vi "ReadWrite Label.vi"(5 "Mode":T10, 6 "ScheduledSDI":bool, 7 "Iteration":i32, 8 "error in (no error)":errorcluster, 10 "FIFOs In":T1, 11 "Label In":T2 {"Driver Data"."Num Bits" min=1 max=32; "Driver Data"."Start Bit" min=8 max=31; "Block Data Refs"."Data Reference" format="%.0x"; "Label" format="%.0o"}) -> (0 "error out":errorcluster, 2 "FIFOs Out":T1, 3 "Label Out":T2 {"Driver Data"."Num Bits" min=1 max=32; "Driver Data"."Start Bit" min=8 max=31; "Block Data Refs"."Data Reference" format="%.0x"; "Label" format="%.0o"})   [LabVIEW 2011, in "AIT 1553 Custom Device.lvlib"]
uses:
  AIT 1553 Custom Device.lvlib
  RT Controls/ReadWrite Selector.ctl
  RT Controls/RT Label Settings.ctl
  Controls and Global/Label.ctl
  Controls and Global/transferPeriod.ctl
  <vilib>/NI Veristand/Custom Device API/Block Data Reference.ctl
  <vilib>/NI Veristand/Custom Device API/Data Reference.ctl
  RT Controls/Driver Data.ctl
  Controls and Global/Start Bit.ctl
  Controls and Global/Number of Bits.ctl
  RT Controls/FIFO.ctl
  Double to selected bits.vi
  SubVIs/Word to double.vi
  <vilib>/NI Veristand/Custom Device API/Global Data Refs.vi
  <instrlib>/AIT 429/Public/Tx/Data/AIT 429 Set Scheduled Label Datum.vi
  <instrlib>/AIT 429/Public/Tx/Data/AIT 429 Get Scheduled Label Datum.vi
  <vilib>/NI Veristand/Custom Device API/Custom Device API.lvlib
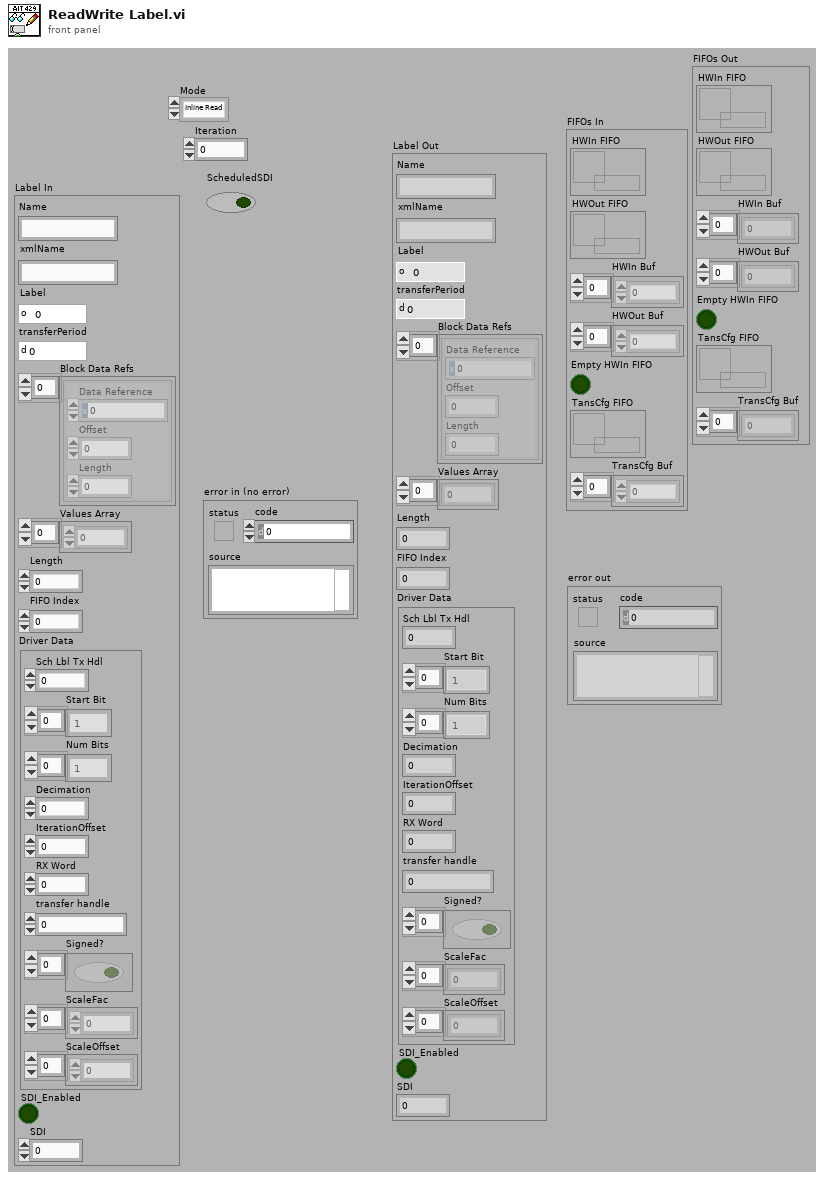
[diagram p1: front panel]
types:
  T1 = typedef "AIT 1553 Custom Device.lvlib/FIFO.ctl" = cluster{"HWIn FIFO":refnum<k33>, "HWOut FIFO":refnum<k33>, "HWIn Buf":dbl[], "HWOut Buf":dbl[], "Empty HWIn FIFO":bool, "TansCfg FIFO":refnum<k33>, "TransCfg Buf":dbl[]}
  T2 = typedef "AIT 1553 Custom Device.lvlib/RT Label Settings.ctl" = cluster{"Name":string, "xmlName":string, "Label":T3, "transferPeriod":T4, "Block Data Refs":T5[], "Values Array":dbl[], "Length":i32, "FIFO Index":i32, "Driver Data":T7, "SDI_Enabled":bool, "SDI":u8}
  T3 = typedef "AIT 1553 Custom Device.lvlib/Label.ctl" = u8
  T4 = typedef "AIT 1553 Custom Device.lvlib/transferPeriod.ctl" = u32
  T5 = typedef "Custom Device API.lvlib/Block Data Reference.ctl" = cluster{"Data Reference":T6, "Offset":i32, "Length":i32}
  T6 = typedef "Custom Device API.lvlib/Data Reference.ctl" = i32
  T7 = typedef "AIT 1553 Custom Device.lvlib/Driver Data.ctl" = cluster{"Sch Lbl Tx Hdl":u32, "Start Bit":T8[], "Num Bits":T9[], "Decimation":i32, "IterationOffset":i32, "RX Word":u32, "transfer handle":u32, "Signed?":bool[], "ScaleFac":dbl[], "ScaleOffset":dbl[]}
  T8 = typedef "AIT 1553 Custom Device.lvlib/Start Bit.ctl" = i32
  T9 = typedef "AIT 1553 Custom Device.lvlib/Number of Bits.ctl" = i32
  T10 = typedef "AIT 1553 Custom Device.lvlib/ReadWrite Selector.ctl" = enum16{"Inline Read", "Inline Write", "Async HWIn", "Async HWOut"}
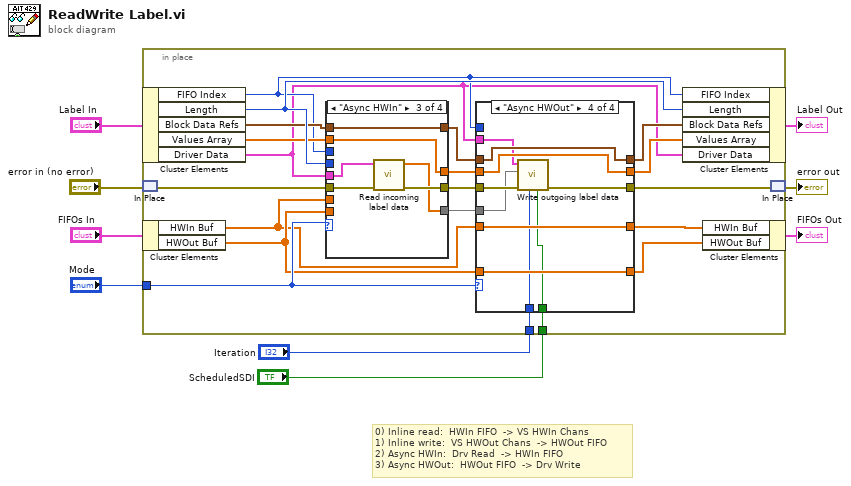
[diagram p0: block diagram]
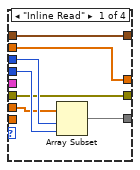
[diagram p2: hidden frame]
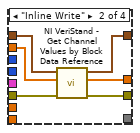
[diagram p3: hidden frame]
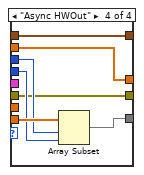
[diagram p4: hidden frame]
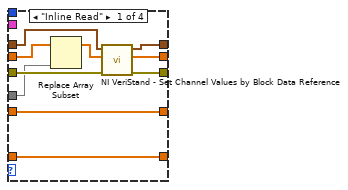
[diagram p5: hidden frame]
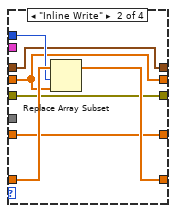
[diagram p6: hidden frame]
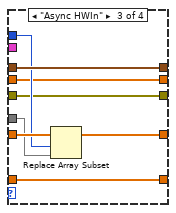
[diagram p7: hidden frame]
diagram:
  # "0) Inline read:\t\tHWIn FIFO \t-> VS HWIn Chans\n1) Inline write: \tVS HWOut Chans \t-> HWOut FIFO\n2) Async HWIn:\t\tDrv Read \t-> HWIn FIFO\n3) Async HWOut: \tHWOut FIFO \t-> Drv Write"
  n1 = in-place {
    in-place-border: "Mode" -> [w29]
    in-place-border: "Iteration" -> [w11]
    in-place-border: "ScheduledSDI" -> [w10]
    n2 = in-place-cluster #1("Label In") -> ("FIFO Index"=w16:i32, "Length"=w24:i32, "Block Data Refs"=w21:T5[], "Values Array"=w20:dbl[], "Driver Data"=w12:T7)
    n3 = in-place-match #2("error in (no error)") -> (w23:errorcluster)
    n4 = in-place-cluster #3("FIFOs In") -> ("HWIn Buf"=w13:dbl[], "HWOut Buf"=w14:dbl[])
    n5 = case shown="\"Async HWIn\"" w29 {
      tunnel: w13 -> [w33 _ _ _]
      tunnel: w16 -> [w36 _ _ w54]
      tunnel: w24 -> [w35 _ _ w53]
      tunnel: [w34 _ w43 w49] -> w28
      tunnel: w23 -> [w30 w42 w46 w50]
      tunnel: [w30 w41 w44 w50] -> w22
      tunnel: w21 -> [w32 w40 w48 w51]
      tunnel: w20 -> [w31 w39 w47 w52]
      tunnel: [w31 w38 w47 w52] -> w18
      tunnel: [w32 w37 w48 w51] -> w19
      tunnel: w12 -> [_ _ w45 _]
      tunnel: w14 -> [_ _ _ w55]
      frame "Inline Read" {
        n6 = Array Subset(array=w33, index=w36, length=w35) -> (w34:dbl[])
      }
      frame "Inline Write" {
        n7 = call <vilib>:"NI VeriStand - Get Channel Values by Block Data Reference.vi"("error in (no error)"=w42, "Values Array in"=w39, "Block Data Ref"=w40) -> ("error out"=w41:errorcluster, "Values Array out"=w38:dbl[], "Block Data Ref dup"=w37:T5[])  [unwired: 6 in]
      }
      frame "Async HWIn" {
        n8 = call "Read incoming label data.vi"("error in (no error)"=w46, "Driver Data"=w45) -> ("error out"=w44:errorcluster, "Values"=w43:dbl[])  [unwired: 8 in]
      }
      frame "Async HWOut" {
        n9 = Array Subset(array=w55, index=w54, length=w53) -> (w49:dbl[])
      }
    }
    n10 = case shown="\"Async HWOut\"" w29 {
      tunnel: w19 -> [w65 w68 w80 w88]
      tunnel: w28 -> [w61 _ w73 w85]
      tunnel: w22 -> [w64 w69 w76 w86]
      tunnel: [w63 w69 w76 w83] -> w27
      tunnel: w18 -> [w62 w67 w74 w87]
      tunnel: [w59 w67 w74 w87] -> w26
      tunnel: [w58 w68 w80 w88] -> w25
      tunnel: w14 -> [w57 w72 w75 w89]
      tunnel: [w57 w71 w75 w89] -> w17
      tunnel: w16 -> [_ w70 w77 _]
      tunnel: w13 -> [w56 w66 w79 w90]
      tunnel: [w56 w66 w78 w90] -> w15
      tunnel: w12 -> [_ _ _ w84]
      tunnel: w11 -> [_ _ _ w82]
      tunnel: w10 -> [_ _ _ w81]
      frame "Inline Read" {
        n11 = Replace Array Subset(array=w62, new element=w61) -> (w60:dbl[])  [unwired: 1 in]
        n12 = call <vilib>:"NI VeriStand - Set Channel Values by Block Data Reference.vi"("error in (no error)"=w64, "Values Array in"=w60, "Block Data Ref"=w65) -> ("error out"=w63:errorcluster, "Values Array out"=w59:dbl[], "Block Data Ref dup"=w58:T5[])  [unwired: 6 in]
      }
      frame "Inline Write" {
        n13 = Replace Array Subset(array=w72, new element=w67, index=w70) -> (w71:dbl[])
      }
      frame "Async HWIn" {
        n14 = Replace Array Subset(array=w79, new element=w73, index=w77) -> (w78:dbl[])
      }
      frame "Async HWOut" {
        n15 = call "Write outgoing label data.vi"("ScheduledSDI"=w81, "Iteration"=w82, "error in (no error)"=w86, "Values"=w85, "Driver Data"=w84) -> ("error out"=w83:errorcluster)  [unwired: 6 in]
      }
    }
    n16 = in-place-cluster #1("FIFO Index"=w16, "Length"=w24, "Block Data Refs"=w25, "Values Array"=w26, "Driver Data"=w12) -> (→"Label Out":T2)
    n17 = in-place-cluster #3("HWIn Buf"=w15, "HWOut Buf"=w17) -> (→"FIFOs Out":T1)
    n18 = in-place-match #2(w27) -> (→"error out":errorcluster)
  }
